vi "Activate or Blackstart Notification.vi"(8 "error in":errorcluster, 10 "Activate or Blackstart":T1, 11 "SCADA in":refnum<class "EMS.lvclass">) -> (0 "error out":errorcluster, 3 "SCADA out":refnum<class "EMS.lvclass">)   [LabVIEW 2018, in "EMS Core.lvlib" / "EMS.lvclass"]
uses:
  EMS.lvclass
  C:/Program Files (x86)/National Instruments/LabVIEW 2018/vi.lib/ActorFramework/Actor/Actor.lvclass
  Optimization/Commissioning Actor/Commissioning/Controls/Activate or Blackstart Selector.ctl
  <vilib>/ActorFramework/Actor/Actor.lvclass/Actor.ctl
  EMS.lvclass/EMS.ctl
  Controls/Microgrid State.ctl
  EMS Messages/Return Microgrid State Msg/Return Microgrid State Msg.lvclass/Return Microgrid State Msg.ctl
  <vilib>/ActorFramework/Message Enqueuer/Message Enqueuer.lvclass/Message Enqueuer.ctl
  <vilib>/ActorFramework/Message Enqueuer/Enqueue.vi
  EMS Messages/Return Microgrid State Msg/Return Microgrid State Msg.lvclass
  C:/Program Files (x86)/National Instruments/LabVIEW 2018/vi.lib/ActorFramework/Message/Message.lvclass
  <vilib>/ActorFramework/Message Priority Queue/Priority Enqueue.vi
  <vilib>/ActorFramework/Actor/Actor.lvclass
  Optimization/Commissioning Actor/Commissioning/Commissioning.lvclass
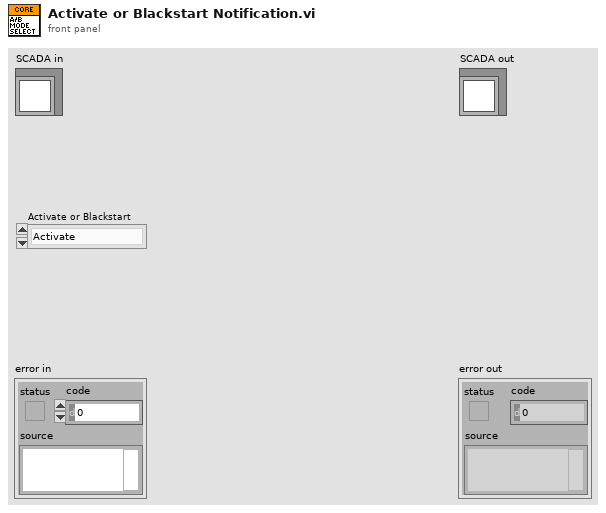
[diagram p1: front panel]
types:
  T1 = typedef "Commissioning Actor.lvlib/Commissioning.lvclass/Activate or Blackstart Selector.ctl" = enum16{"Activate", "Blackstart"}
  T2 = typedef "EMS Core.lvlib/EMS.lvclass/Microgrid State.ctl" = enum16{"Discovery", "Commissioning", "Activation", "Blackstart", "OnGrid", "OffGrid", "Island", "Resynchronization", "Manual", "Shutdown", "Stop"}
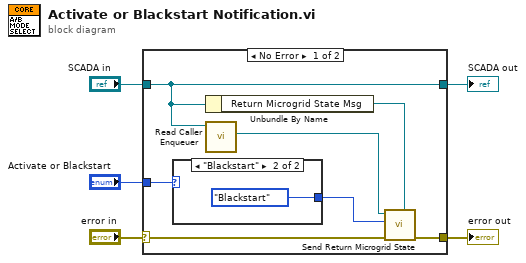
[diagram p0: block diagram]
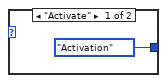
[diagram p2: hidden frame]
diagram:
  n1 = case shown="No Error" "error in" {
    selector: "error in" -> [w7 w16]
    tunnel: [w6 w16] -> w4
    tunnel: [w12 w15] -> w2
    tunnel: "SCADA in" -> [w12 w15]
    tunnel: "Activate or Blackstart" -> [w9 _]
    frame No Error {
      n2 = case shown="\"Blackstart\"" w9 {
        tunnel: [Microgrid_State."Activation" ("Microgrid State") Microgrid_State."Blackstart" ("Microgrid State")] -> w8
        frame "Activate" {
        }
        frame "Blackstart" {
        }
      }
      n3 = Unbundle By Name(w12) -> ("Return Microgrid State Msg"=w11:refnum<class "Return Microgrid State Msg.lvclass">)
      n4 = call <vilib>:"Read Caller Enqueuer.vi"("Actor"=w12) -> ("Caller Enqueuer"=w10:refnum<class "Message Enqueuer.lvclass">)  [unwired: 10 in]
      n5 = call "Send Return Microgrid State.vi"("Message Type"=w11, "error in (no error)"=w7, "Microgrid State"=w8, "Message Enqueuer"=w10) -> ("error out"=w6:errorcluster)  [unwired: 6 in, 1 out]
    }
    frame Error {
    }
  }
  "error out" <- w4
  "SCADA out" <- w2
